vi "Param (SubVI).vi"(6 "Удалить кавычки":bool=TRUE, 8 "error in":errorcluster, 9 "Item":string, 10 "Param":string, 11 "<JSON>":string) -> (0 "error out":errorcluster, 3 "Array":string[](array[string]))   [LabVIEW 2017, in "LV_Unicorn.lvlib"]
uses:
  LV_Unicorn.lvlib
  <vilib>/JDP Science/JSONtext/Next JSON Value.vi
  <vilib>/JDP Science/JSONtext/String Subset.vi
  <vilib>/JDP Science/JSONtext/Parsing/Advance past next JSON Value (inlined COPY).vi
  <vilib>/JDP Science/JSONtext/Parsing/Advance past whitespace.vi
  <vilib>/JDP Science/JSONtext/Parsing/Advance past String.vi
  <vilib>/JDP Science/JSONtext/Parsing/Advance past Number.vi
  <vilib>/JDP Science/JSONtext/Parsing/Advance past Line Ending.vi
  <vilib>/JDP Science/JSONtext/Parsing/Parse Full Path or Item Name.vi
  <vilib>/JDP Science/JSONtext/Parsing/Advance past Array.vi
  <vilib>/JDP Science/JSONtext/Parsing/Advance past Object.vi
  <vilib>/JDP Science/JSONtext/support/Error Cluster From Code.vi
  <vilib>/JDP Science/JSONtext/Offset/Find Item Locations by Path.vi
  <vilib>/JDP Science/JSONtext/JSONtext.lvlib
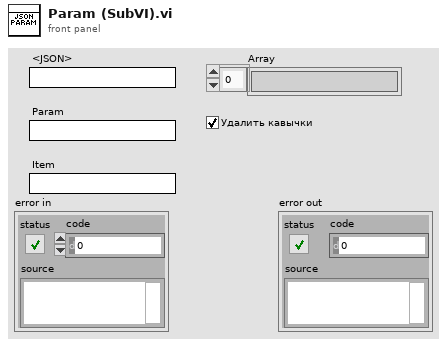
[diagram p1: front panel]
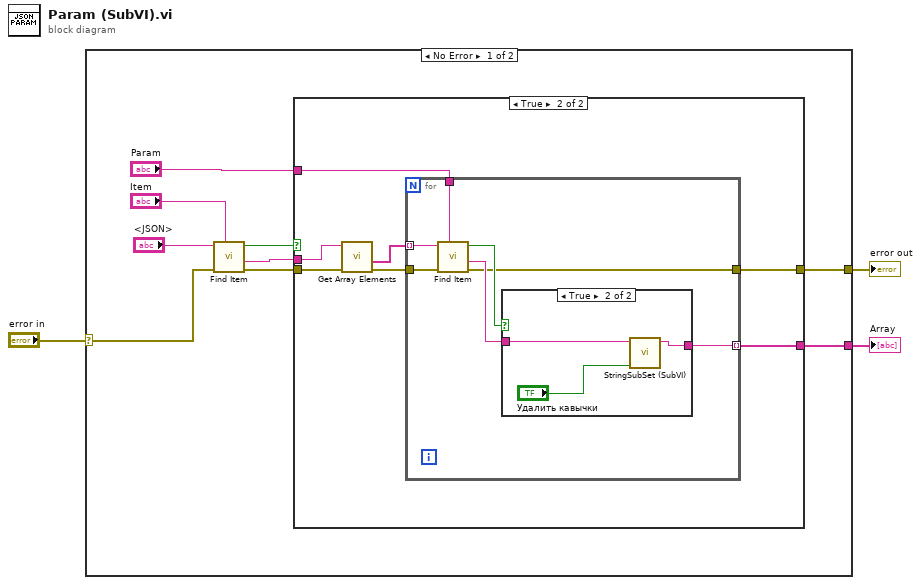
[diagram p0: block diagram]
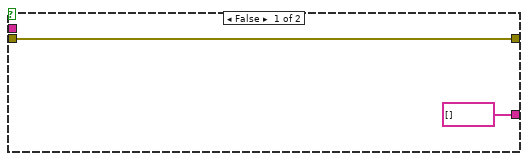
[diagram p2: hidden frame]
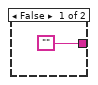
[diagram p3: hidden frame]
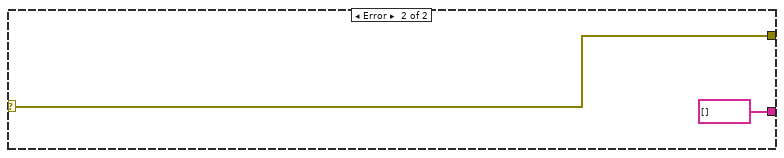
[diagram p4: hidden frame]
diagram:
  n1 = case shown="No Error" "error in" {
    selector: "error in" -> [w4 w34]
    tunnel: [w11 string[] []] -> w3
    tunnel: [w5 w34] -> w2
    frame No Error {
      n2 = call <vilib>:"Find Item.vi"("$Path or Item Name"="Item", "error in (no error)"=w4, "JSON"="<JSON>") -> ("error out"=w6:errorcluster, "<JSON>"=w8:string, "Found"=w10:bool)  [unwired: 5 in, 1 out]
      n3 = case shown="True" w10 {
        tunnel: w8 -> [_ w21]
        tunnel: [string[] [] w19] -> w11
        tunnel: "Param" -> [_ w18]
        tunnel: w6 -> [w14 w17]
        tunnel: [w14 w15] -> w5
        frame False {
        }
        frame True {
          n4 = call <vilib>:"Get Array Elements.vi"("error in (no error)"=w17, "JSON"=w21) -> ("error out"=w16:errorcluster, "<JSON>"=w20:string[])  [unwired: 7 in, 1 out]
          n5 = for {
            tunnel: w20 -> [w28] mode=indexing
            tunnel: [w26] -> w19 mode=indexing
            tunnel: w18 -> [w24]
            tunnel: w16 -> [w23]
            tunnel: [w22] -> w15
            n6 = call <vilib>:"Find Item.vi"("$Path or Item Name"=w24, "error in (no error)"=w23, "JSON"=w28) -> ("error out"=w22:errorcluster, "<JSON>"=w27:string, "Found"=w25:bool)  [unwired: 5 in, 1 out]
            n7 = case shown="True" w25 {
              tunnel: w27 -> [_ w32]
              tunnel: ["" w31] -> w26
              frame False {
              }
              frame True {
                n8 = call "StringSubSet (SubVI).vi"("Удалить кавычки"="Удалить кавычки", "<JSON> in"=w32) -> ("<JSON> out"=w31:string)  [unwired: 9 in]
              }
            }
          }
        }
      }
    }
    frame Error {
    }
  }
  "Array" <- w3
  "error out" <- w2
